vi "convert scan cluster to file scan with drift check.vi"(0 "Scan parameters":T1 {"Scan Start" format="%#.9p"; "Scan End" format="%#.9p"; "Scan Step Size" format="%#.9p"}, 1 "check value":dbl, 2 "precision (12)":i16=12) -> (7 "spreadsheet string":string, 8 "values":string[](array[string]), 9 "values:numshots":string[](array[string]))   [LabVIEW 2013]
uses:
  scan parameters.ctl
  <vilib>/Analysis/1siggen.llb/Ramp Pattern by Delta.vi
  <vilib>/Analysis/NI_AALBase.lvlib
panel:
  out "Ramp Pattern":dbl[](array[numeric])
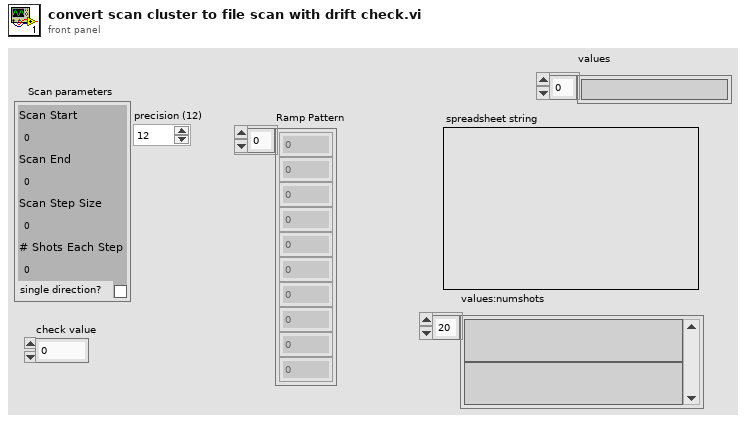
[diagram p1: front panel]
types:
  T1 = typedef "scan parameters.ctl" = cluster{"Scan Start":dbl, "Scan End":dbl, "Scan Step Size":dbl, "# Shots Each Step":u32, "single direction?":bool}
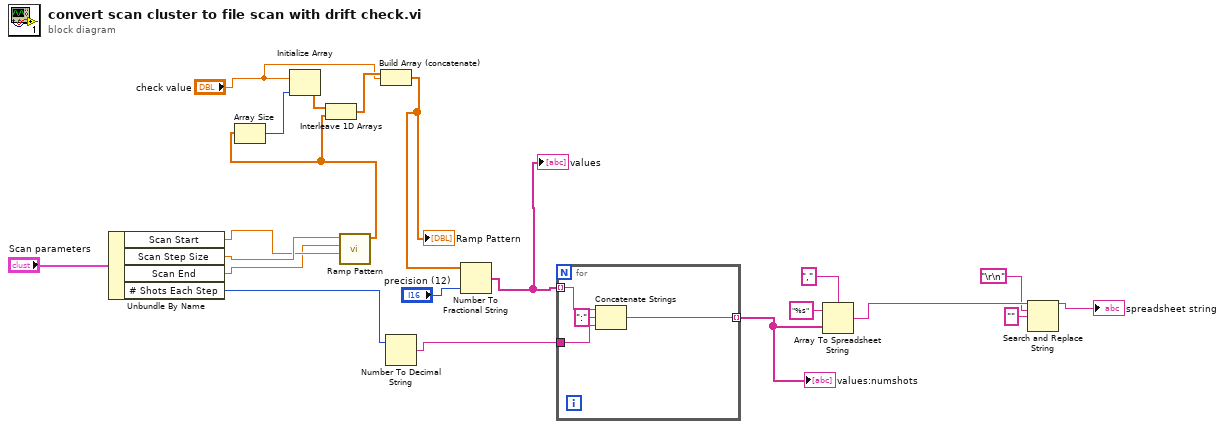
[diagram p0: block diagram]
diagram:
  n1 = Unbundle By Name("Scan parameters") -> ("Scan Start"=w19:dbl, "Scan Step Size"=w20:dbl, "Scan End"=w18:dbl, "# Shots Each Step"=w16:u32)
  n2 = call-poly <vilib>:"Ramp Pattern.vi"("start"=w19, "end"=w18, "delta"=w20) -> ("Ramp Pattern"=w6:dbl[])  [unwired: 6 in, 2 out]
  n3 = Array Size(array=w6) -> (size(s)=w5:i32)
  n4 = Initialize Array("check value", w5) -> (w4:dbl[])
  n5 = Interleave 1D Arrays(w4, w6) -> (w3:dbl[])
  n6 = Build Array (concatenate)(w3, "check value") -> (w1:dbl[])
  "Ramp Pattern" <- w1
  n7 = Number To Decimal String(number=w16) -> (decimal integer string=w15:string)  [unwired: 1 in]
  n8 = Number To Fractional String(number=w1, precision (6)="precision (12)") -> (F-format string=w11:string[])  [unwired: 2 in]
  "values" <- w11
  n9 = for {
    tunnel: w11 -> [w25] mode=indexing
    tunnel: w15 -> [w23]
    tunnel: [w22] -> w14 mode=indexing
    n10 = Concatenate Strings(w25, ":" ("string"), w23) -> (w22:string)
  }
  "values:numshots" <- w14
  n11 = Array To Spreadsheet String(delimiter (Tab)=",", array=w14, 3:"%s" ("format string")) -> (spreadsheet string=w10:string)
  n12 = Search and Replace String(input string=w10, search string="\r\n", replace string="" ("replace string (\"\")")) -> (result string=→"spreadsheet string":string)  [unwired: 5 in, 3 out]
